vi "Ev o.vi"(8 "error in (no error)":errorcluster, 11 "IDE simple in":refnum<class "Main Panel.lvclass">) -> (0 "error out":errorcluster, 3 "IDE simple out":refnum<class "Main Panel.lvclass">)   [LabVIEW 2018, in "Main Panel.lvlib" / "Main Panel.lvclass"]
uses:
  Main Panel.lvclass
  Main Panel.lvclass/Main Panel.ctl
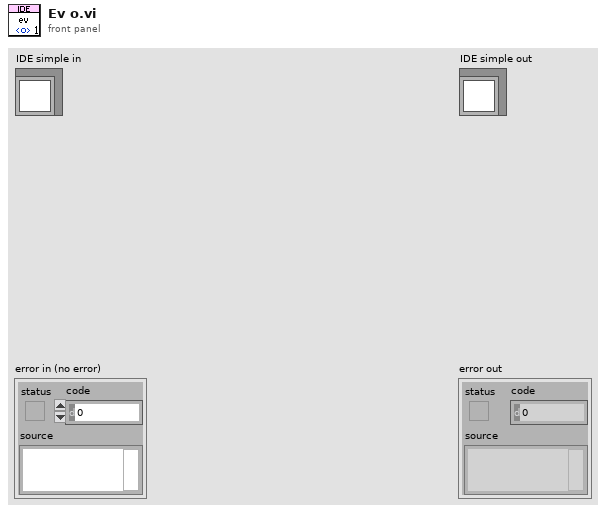
[diagram p1: front panel]
types:
  T1 = typedef "Data Parser.lvclass/frame o data.ctl" = cluster{"kind":string, "x":string, "y":string, "action":string, "dvx":string, "dvy":string, "dvz":string, "oid":string, "facing":string}
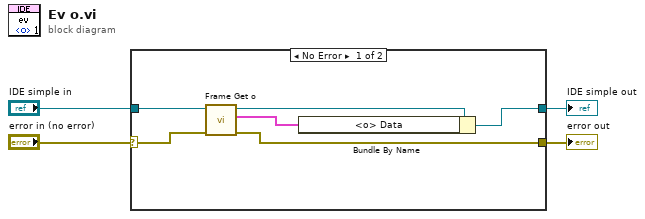
[diagram p0: block diagram]
diagram:
  n1 = case shown="No Error" "error in (no error)" {
    selector: "error in (no error)" -> [w9 w12]
    tunnel: [w6 w12] -> w3
    tunnel: [w5 w11] -> w1
    tunnel: "IDE simple in" -> [w10 w11]
    frame No Error {
      n2 = call "Frame Get o.vi"("error in (no error)"=w9, "IDE simple in"=w10) -> ("error out"=w6:errorcluster, "<o> Data"=w7:T1, "IDE simple out"=w8:refnum<class "Main Panel.lvclass">)  [unwired: 7 in]
      n3 = Bundle By Name(cluster=w8, "<o> Data"=w7) -> (w5:refnum<class "Main Panel.lvclass">)
    }
    frame Error {
    }
  }
  "error out" <- w3
  "IDE simple out" <- w1
